vi "Read Service ID.vi"(8 "error in (no error)":errorcluster, 11 "Room Service Monitor UI in":refnum<class "Room Service Monitor UI.lvclass">) -> (0 "error out":errorcluster, 2 "Service ID":string, 3 "Room Service Monitor UI out":refnum<class "Room Service Monitor UI.lvclass">)   [LabVIEW 2023, in "Room Service Monitor UI.lvlib" / "Room Service Monitor UI.lvclass"]
uses:
  Room Service Monitor UI.lvclass
  Room Service Monitor UI.lvclass/Room Service Monitor UI.ctl
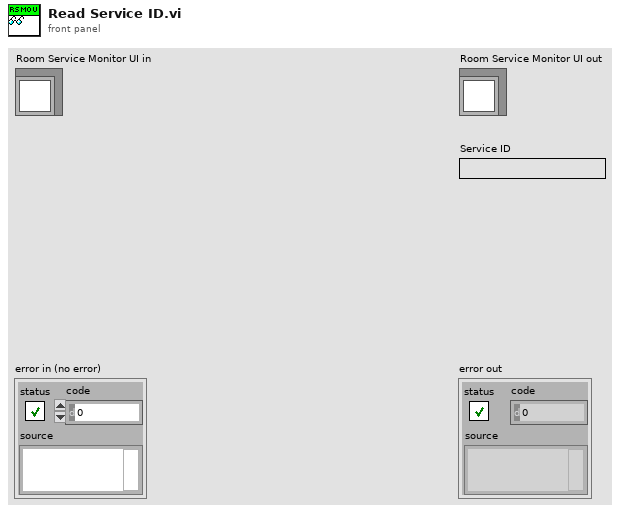
[diagram p1: front panel]
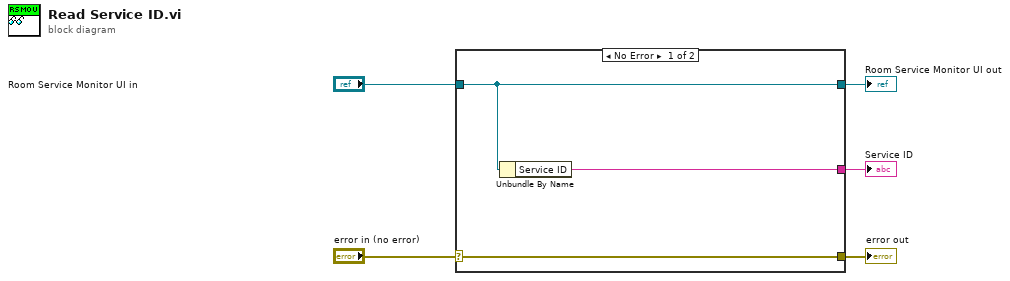
[diagram p0: block diagram]
diagram:
  n1 = case shown="No Error" "error in (no error)" {
    selector: "error in (no error)" -> [w8 w9]
    tunnel: [w8 w9] -> w4
    tunnel: [w7 w10] -> w2
    tunnel: "Room Service Monitor UI in" -> [w7 w10]
    tunnel: [w6 _] -> w1
    frame No Error {
      n2 = Unbundle By Name(w7) -> ("Service ID"=w6:string)
    }
    frame Error {
    }
  }
  "error out" <- w4
  "Room Service Monitor UI out" <- w2
  "Service ID" <- w1
